vi "modified_data_server_example.vi"() -> ()   [LabVIEW 2013, in "TCP_IP.lvclass"]
doc: "Sends a specified waveform through a TCP port. The VI first listens for a connection and, once established, sends the number of bytes to be sent followed by the data. After the data is sent, the VI waits for an 'all received' signal from the client and then breaks the connection.\n\n<B>Note:</B> Requires the Data Client.vi located in the same library as this VI."
uses:
  TCP_IP.lvclass
panel:
  in  "amplitude period (ms)":u32
  out "Waveform Graph":dbl[](graph)
  out "*(type *) &x":string
  out "remote address":string
  in  "stop":bool
  in  "Noise Level":dbl(slide)=0.36734693877551017 scale=0.0..1.0 scale format="%0.1f"
  in  "# of Points":i32=200
  in  "Function":u16(ring)=1 items=["random", "sine wave", "cosine wave"]
  in  "Port":u16=6340 min=1025 step=1
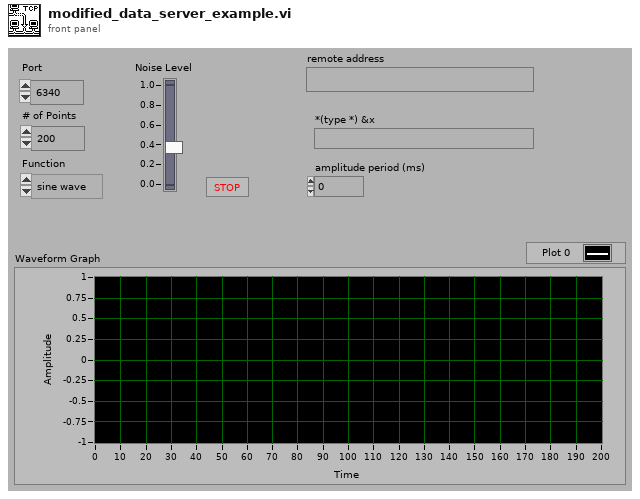
[diagram p1: front panel]
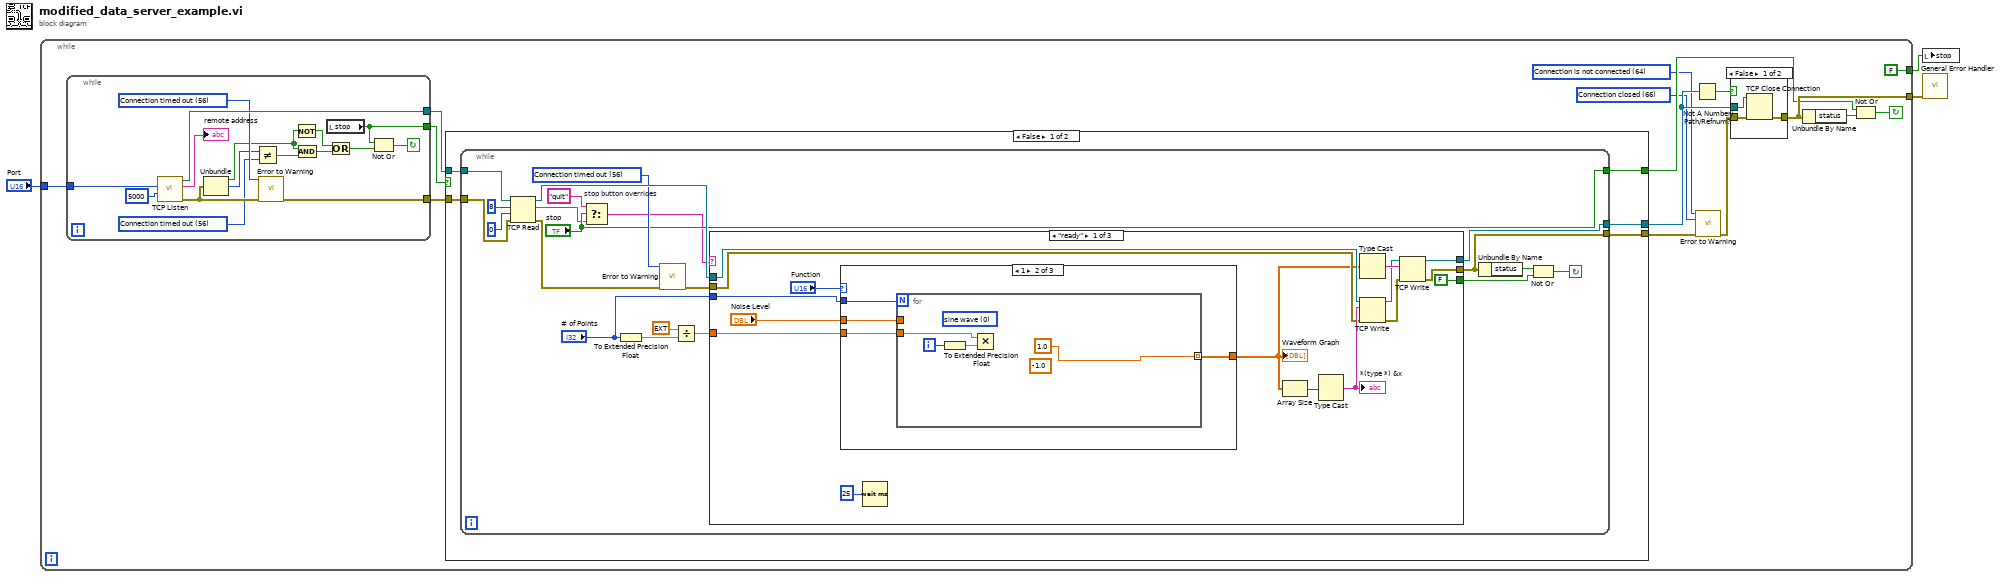
[diagram p0: block diagram]
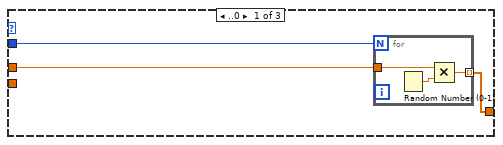
[diagram p2: hidden frame]
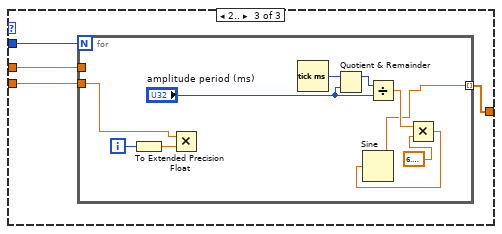
[diagram p3: hidden frame]
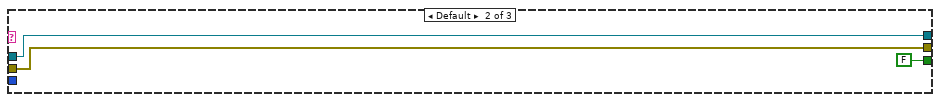
[diagram p4: hidden frame]
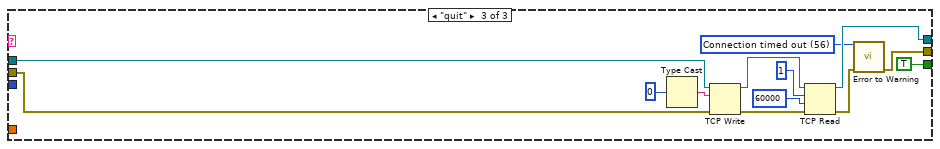
[diagram p5: hidden frame]
diagram:
  n1 = while {
    tunnel: [w11] -> w2
    tunnel: "Port" -> [w17]
    tunnel: [FALSE] -> w1
    stop <- w18 continue-if-true
    w6 = 66 items=["No Error", "Argument Error", "Memory Full", "Out of Zone", "End of File", "File Already Open", "Generic File IO Error", "File Not Found", "File Permission Error", "Disk Full", "Duplicate Path", "Too Many Files Open", "Not Enabled", "Resource File Not Found", "Cannot Add Resource", "Resource Not Found", "Image Not Found", "Image Memory Error", "Pen Does Not Exist", "Config Bad Type", "Config Token Not Found", "Config Parse Error", "Config Memory Error", "Bad External Code Format", "Bad External Code Offset", "External Code Not Present", "Null Window", "Destroy Window Mixup", "Null Menu", "Print Aborted", "Bad Print Record", "Print Driver Error", "Windows Error During Print", "Memory Error During Print", "Print Dialog Error", "Generic Print Error", "Invalid Device Refnum", "Device Not Found", "Device Parameter Error", "Device Unit Error", "Can't Open Device", "Device Call Aborted", "Generic Error", "Cancelled By User", "Object ID Too Low", "Object ID Too High", "Object Not In Heap", "Unknown Heap", "Bad DefProc ID", "DefProc Not In Table", "Message Out Of Range", "Null Method", "Unknown Message", "Manager Call Not Supported", "Bad address", "Connection In progress", "Connection timed out", "Connection is already in progress", "Network attribute not supported", "Network error", "Address in use", "System out of memory", "Connection aborted", "Connection refused", "Connection is not connected", "Connection is already connected", "Connection closed", "Initialize error (interapplication manager)", "Bad occurrence", "Wait on unbound occurrence handler", "Occurrence queue overflow", "Bad path", "Semaphore not signaled", "Unrecognized type (interapplication manager)"] ("2nd Error to Convert")
    w7 = 64 items=["No Error", "Argument Error", "Memory Full", "Out of Zone", "End of File", "File Already Open", "Generic File IO Error", "File Not Found", "File Permission Error", "Disk Full", "Duplicate Path", "Too Many Files Open", "Not Enabled", "Resource File Not Found", "Cannot Add Resource", "Resource Not Found", "Image Not Found", "Image Memory Error", "Pen Does Not Exist", "Config Bad Type", "Config Token Not Found", "Config Parse Error", "Config Memory Error", "Bad External Code Format", "Bad External Code Offset", "External Code Not Present", "Null Window", "Destroy Window Mixup", "Null Menu", "Print Aborted", "Bad Print Record", "Print Driver Error", "Windows Error During Print", "Memory Error During Print", "Print Dialog Error", "Generic Print Error", "Invalid Device Refnum", "Device Not Found", "Device Parameter Error", "Device Unit Error", "Can't Open Device", "Device Call Aborted", "Generic Error", "Cancelled By User", "Object ID Too Low", "Object ID Too High", "Object Not In Heap", "Unknown Heap", "Bad DefProc ID", "DefProc Not In Table", "Message Out Of Range", "Null Method", "Unknown Message", "Manager Call Not Supported", "Bad address", "Connection In progress", "Connection timed out", "Connection is already in progress", "Network attribute not supported", "Network error", "Address in use", "System out of memory", "Connection aborted", "Connection refused", "Connection is not connected", "Connection is already connected", "Connection closed", "Initialize error (interapplication manager)", "Bad occurrence", "Wait on unbound occurrence handler", "Occurrence queue overflow", "Bad path", "Semaphore not signaled", "Unrecognized type (interapplication manager)"] ("1st Error to Convert")
    n2 = while {
      tunnel: [w20] -> w14
      tunnel: [w29] -> w15
      tunnel: [w33] -> w16
      tunnel: w17 -> [w34]
      stop <- w31 continue-if-true
      w27 = 56 items=["No Error", "Argument Error", "Memory Full", "Out of Zone", "End of File", "File Already Open", "Generic File IO Error", "File Not Found", "File Permission Error", "Disk Full", "Duplicate Path", "Too Many Files Open", "Not Enabled", "Resource File Not Found", "Cannot Add Resource", "Resource Not Found", "Image Not Found", "Image Memory Error", "Pen Does Not Exist", "Config Bad Type", "Config Token Not Found", "Config Parse Error", "Config Memory Error", "Bad External Code Format", "Bad External Code Offset", "External Code Not Present", "Null Window", "Destroy Window Mixup", "Null Menu", "Print Aborted", "Bad Print Record", "Print Driver Error", "Windows Error During Print", "Memory Error During Print", "Print Dialog Error", "Generic Print Error", "Invalid Device Refnum", "Device Not Found", "Device Parameter Error", "Device Unit Error", "Can't Open Device", "Device Call Aborted", "Generic Error", "Cancelled By User", "Object ID Too Low", "Object ID Too High", "Object Not In Heap", "Unknown Heap", "Bad DefProc ID", "DefProc Not In Table", "Message Out Of Range", "Null Method", "Unknown Message", "Manager Call Not Supported", "Bad address", "Connection In progress", "Connection timed out", "Connection is already in progress", "Network attribute not supported", "Network error", "Address in use", "System out of memory", "Connection aborted", "Connection refused", "Connection is not connected", "Connection is already connected", "Connection closed", "Initialize error (interapplication manager)", "Bad occurrence", "Wait on unbound occurrence handler", "Occurrence queue overflow", "Bad path", "Semaphore not signaled", "Unrecognized type (interapplication manager)"] ("1st Error to Convert")
      w28 = 56 items=["No Error", "Argument Error", "Memory Full", "Out of Zone", "End of File", "File Already Open", "Generic File IO Error", "File Not Found", "File Permission Error", "Disk Full", "Duplicate Path", "Too Many Files Open", "Not Enabled", "Resource File Not Found", "Cannot Add Resource", "Resource Not Found", "Image Not Found", "Image Memory Error", "Pen Does Not Exist", "Config Bad Type", "Config Token Not Found", "Config Parse Error", "Config Memory Error", "Bad External Code Format", "Bad External Code Offset", "External Code Not Present", "Null Window", "Destroy Window Mixup", "Null Menu", "Print Aborted", "Bad Print Record", "Print Driver Error", "Windows Error During Print", "Memory Error During Print", "Print Dialog Error", "Generic Print Error", "Invalid Device Refnum", "Device Not Found", "Device Parameter Error", "Device Unit Error", "Can't Open Device", "Device Call Aborted", "Generic Error", "Cancelled By User", "Object ID Too Low", "Object ID Too High", "Object Not In Heap", "Unknown Heap", "Bad DefProc ID", "DefProc Not In Table", "Message Out Of Range", "Null Method", "Unknown Message", "Manager Call Not Supported", "Bad address", "Connection In progress", "Connection timed out", "Connection is already in progress", "Network attribute not supported", "Network error", "Address in use", "System out of memory", "Connection aborted", "Connection refused", "Connection is not connected", "Connection is already connected", "Connection closed", "Initialize error (interapplication manager)", "Bad occurrence", "Wait on unbound occurrence handler", "Occurrence queue overflow", "Bad path", "Semaphore not signaled", "Unrecognized type (interapplication manager)"] ("1st Error to Convert")
      n3 = call <vilib>:"TCP Listen.vi"("timeout ms (wait forever: -1)"=5000, "port"=w34) -> ("error out"=w30:errorcluster, "remote address"=→"remote address":string, "connection ID"=w33:refnum<k5>)  [unwired: 5 in, 2 out]
      n4 = Unbundle(w30) -> ("status"=w25:bool, "code"=w26:i32)  [unwired: 1 out]
      n5 = Not Equal?(x=w26, y=w27) -> (x != y?=w24:bool)
      n6 = call <vilib>:"Error to Warning.vi"("1st Error to Convert"=w28, "error in"=w30) -> ("warning out"=w29:errorcluster)  [unwired: 13 in]
      n7 = Not(x=w25) -> (.not. x?=w23:bool)
      n8 = And(x=w25, y=w24) -> (x .and. y?=w22:bool)
      n9 = local read "stop"() -> (w20:bool)
      n10 = Or(x=w23, y=w22) -> (x .or. y?=w21:bool)
      n11 = Not Or(1:w21, 2:w20) -> (0:w31:bool)
    }
    n12 = case shown="False" w14 {
      selector: w14 -> [_ w121]
      tunnel: [w39 w122] -> w5
      tunnel: w16 -> [w38 w123]
      tunnel: w15 -> [w37 w122]
      tunnel: [w36 w123] -> w13
      tunnel: [w35 w121] -> w9
      frame False {
        n13 = while {
          tunnel: ["stop"] -> w35
          tunnel: w37 -> [w57]
          tunnel: [w52] -> w39
          tunnel: [w54] -> w36
          tunnel: w38 -> [w56]
          stop <- w60 continue-if-true
          w46 = 56 items=["No Error", "Argument Error", "Memory Full", "Out of Zone", "End of File", "File Already Open", "Generic File IO Error", "File Not Found", "File Permission Error", "Disk Full", "Duplicate Path", "Too Many Files Open", "Not Enabled", "Resource File Not Found", "Cannot Add Resource", "Resource Not Found", "Image Not Found", "Image Memory Error", "Pen Does Not Exist", "Config Bad Type", "Config Token Not Found", "Config Parse Error", "Config Memory Error", "Bad External Code Format", "Bad External Code Offset", "External Code Not Present", "Null Window", "Destroy Window Mixup", "Null Menu", "Print Aborted", "Bad Print Record", "Print Driver Error", "Windows Error During Print", "Memory Error During Print", "Print Dialog Error", "Generic Print Error", "Invalid Device Refnum", "Device Not Found", "Device Parameter Error", "Device Unit Error", "Can't Open Device", "Device Call Aborted", "Generic Error", "Cancelled By User", "Object ID Too Low", "Object ID Too High", "Object Not In Heap", "Unknown Heap", "Bad DefProc ID", "DefProc Not In Table", "Message Out Of Range", "Null Method", "Unknown Message", "Manager Call Not Supported", "Bad address", "Connection In progress", "Connection timed out", "Connection is already in progress", "Network attribute not supported", "Network error", "Address in use", "System out of memory", "Connection aborted", "Connection refused", "Connection is not connected", "Connection is already connected", "Connection closed", "Initialize error (interapplication manager)", "Bad occurrence", "Wait on unbound occurrence handler", "Occurrence queue overflow", "Bad path", "Semaphore not signaled", "Unrecognized type (interapplication manager)"] ("1st Error to Convert")
          n14 = TCP Read(connection ID=w56, bytes to read=8, error in (no error)=w57, 9:0) -> (connection ID out=w55:refnum<k5>, data out=w41:string, error out=w45:errorcluster)  [unwired: 1 in]
          n15 = Select "stop button overrides"(t="quit", s="stop", f=w41) -> (s? t:f=w40:string)
          n16 = To Extended Precision Float(1:"# of Points") -> (0:w50:ext)
          n17 = call <vilib>:"Error to Warning.vi"("1st Error to Convert"=w46, "error in"=w45) -> ("warning out"=w44:errorcluster)  [unwired: 13 in]
          n18 = Divide(x=ext 6.283185307179586477, y=w50) -> (x/y=w47:ext)
          n19 = case shown="\"ready\"" w40 {
            tunnel: w44 -> [w72 w107 w116]
            tunnel: w55 -> [w71 w106 w114]
            tunnel: [w70 w106 w118] -> w54
            tunnel: [w69 w107 w109] -> w52
            tunnel: [FALSE FALSE TRUE] -> w53
            tunnel: "# of Points" -> [w65 _ _]
            tunnel: w47 -> [w64 _ _]
            frame "ready" {
              n20 = case shown="1" "Function" {
                tunnel: w65 -> [w79 w86 w94]
                tunnel: [w78 w83 w91] -> w62
                tunnel: w64 -> [_ w85 w92]
                tunnel: "Noise Level" -> [w77 w84 w93]
                frame ..0 {
                  n21 = for {
                    N: w79 -> [_]
                    tunnel: [w80] -> w78 mode=indexing
                    tunnel: w77 -> [w82]
                    n22 = Random Number (0-1)() -> (number: 0 to 1=w81:dbl)
                    n23 = Multiply(x=w82, y=w81) -> (x*y=w80:dbl)
                  }
                }
                frame 1 {
                  n24 = for {
                    N: w86 -> [_]
                    tunnel: w85 -> [w89]
                    tunnel: w84 -> [_]
                    tunnel: [1.0] -> w83 mode=indexing
                    i -> [w90]
                    (unwired) u16 0 items=["sine wave", "cosine wave"] ("Function")
                    (unwired) -1.0
                    n25 = To Extended Precision Float(1:w90) -> (0:w88:ext)
                    n26 = Multiply(x=w89, y=w88) -> ()  [unwired: 1 out]
                  }
                }
                frame 2.. {
                  n27 = for {
                    N: w94 -> [_]
                    tunnel: w93 -> [_]
                    tunnel: w92 -> [w102]
                    tunnel: [w95] -> w91 mode=indexing
                    i -> [w104]
                    n28 = To Extended Precision Float(1:w104) -> (0:w103:ext)
                    n29 = Multiply(x=w102, y=w103) -> ()  [unwired: 1 out]
                    n30 = Tick Count (ms)() -> (millisecond timer value=w101:u32)
                    n31 = Quotient & Remainder(x=w101, y="amplitude period (ms)") -> (x-y*floor(x/y)=w100:u32)  [unwired: 1 out]
                    n32 = Divide(x=w100, y="amplitude period (ms)") -> (x/y=w98:dbl)
                    n33 = Multiply(x=w98, y=6.283185307179586) -> (x*y=w96:dbl)
                    n34 = Sine(x=w96) -> (sin(x)=w95:dbl)
                  }
                }
              }
              "Waveform Graph" <- w62
              n35 = Wait (ms)(milliseconds to wait=u32 25) -> ()  [unwired: 1 out]
              n36 = Array Size(array=w62) -> (size(s)=w61:i32)
              n37 = Type Cast(x=w61) -> (*(type *) &x=w75:string)  [unwired: 1 in]
              "*(type *) &x" <- w75
              n38 = Type Cast(x=w62) -> (*(type *) &x=w76:string)  [unwired: 1 in]
              n39 = TCP Write(connection ID=w71, data in=w75, error in (no error)=w72) -> (connection ID out=w73:refnum<k5>, error out=w74:errorcluster)  [unwired: 1 in, 1 out]
              n40 = TCP Write(connection ID=w73, data in=w76, error in (no error)=w74) -> (connection ID out=w70:refnum<k5>, error out=w69:errorcluster)  [unwired: 1 in, 1 out]
            }
            frame Default {
            }
            frame "quit" {
              w108 = 56 items=["No Error", "Argument Error", "Memory Full", "Out of Zone", "End of File", "File Already Open", "Generic File IO Error", "File Not Found", "File Permission Error", "Disk Full", "Duplicate Path", "Too Many Files Open", "Not Enabled", "Resource File Not Found", "Cannot Add Resource", "Resource Not Found", "Image Not Found", "Image Memory Error", "Pen Does Not Exist", "Config Bad Type", "Config Token Not Found", "Config Parse Error", "Config Memory Error", "Bad External Code Format", "Bad External Code Offset", "External Code Not Present", "Null Window", "Destroy Window Mixup", "Null Menu", "Print Aborted", "Bad Print Record", "Print Driver Error", "Windows Error During Print", "Memory Error During Print", "Print Dialog Error", "Generic Print Error", "Invalid Device Refnum", "Device Not Found", "Device Parameter Error", "Device Unit Error", "Can't Open Device", "Device Call Aborted", "Generic Error", "Cancelled By User", "Object ID Too Low", "Object ID Too High", "Object Not In Heap", "Unknown Heap", "Bad DefProc ID", "DefProc Not In Table", "Message Out Of Range", "Null Method", "Unknown Message", "Manager Call Not Supported", "Bad address", "Connection In progress", "Connection timed out", "Connection is already in progress", "Network attribute not supported", "Network error", "Address in use", "System out of memory", "Connection aborted", "Connection refused", "Connection is not connected", "Connection is already connected", "Connection closed", "Initialize error (interapplication manager)", "Bad occurrence", "Wait on unbound occurrence handler", "Occurrence queue overflow", "Bad path", "Semaphore not signaled", "Unrecognized type (interapplication manager)"] ("1st Error to Convert")
              n41 = Type Cast(x=0) -> (*(type *) &x=w111:string)  [unwired: 1 in]
              n42 = TCP Write(connection ID=w114, data in=w111, error in (no error)=w116) -> (connection ID out=w113:refnum<k5>, error out=w115:errorcluster)  [unwired: 1 in, 1 out]
              n43 = TCP Read(connection ID=w113, bytes to read=1, error in (no error)=w115, 9:60000) -> (connection ID out=w118:refnum<k5>, error out=w110:errorcluster)  [unwired: 1 in, 1 out]
              n44 = call <vilib>:"Error to Warning.vi"("1st Error to Convert"=w108, "error in"=w110) -> ("warning out"=w109:errorcluster)  [unwired: 13 in]
            }
          }
          n45 = Unbundle By Name(w52) -> ("status"=w51:bool)
          n46 = Not Or(1:w53, 2:w51) -> (0:w60:bool)
        }
      }
      frame True {
      }
    }
    n47 = Not A Number/Path/Refnum?(number/path/refnum=w13) -> (NaN/Path/Refnum?=w12:bool)
    n48 = call <vilib>:"Error to Warning.vi"("1st Error to Convert"=w7, "2nd Error to Convert"=w6, "error in"=w5) -> ("warning out"=w4:errorcluster)  [unwired: 12 in]
    n49 = case shown="False" w12 {
      tunnel: w4 -> [w126 w127]
      tunnel: w13 -> [w125 _]
      tunnel: [w124 w127] -> w11
      frame False {
        n50 = TCP Close Connection(connection ID=w125, error in (no error)=w126) -> (error out=w124:errorcluster)  [unwired: 1 in, 1 out]
      }
      frame True {
      }
    }
    n51 = Unbundle By Name(w11) -> ("status"=w10:bool)
    n52 = Not Or(1:w10, 2:w9) -> (0:w18:bool)
  }
  n53 = local write "stop"(w1) -> ()
  n54 = call <vilib>:"General Error Handler.vi"("error in (no error)"=w2) -> ()  [unwired: 10 in, 5 out]
